vi "init.vi"(8 "error in (no error)":errorcluster, 11 "Counter in":refnum<class "Counter.lvclass">) -> (0 "error out":errorcluster, 3 "Counter out":refnum<class "Counter.lvclass">)   [LabVIEW 2014, in "Counter.lvclass"]
uses:
  Counter.lvclass
  Counter.lvclass/Counter.ctl
  Globals.vi
  <vilib>/DAQmx/create/channels.llb/DAQmx Create Channel (CI-Count Edges).vi
  <vilib>/DAQmx/configure/timing.llb/DAQmx Timing (Sample Clock).vi
  <resource>/objmgr/daqmx.rc
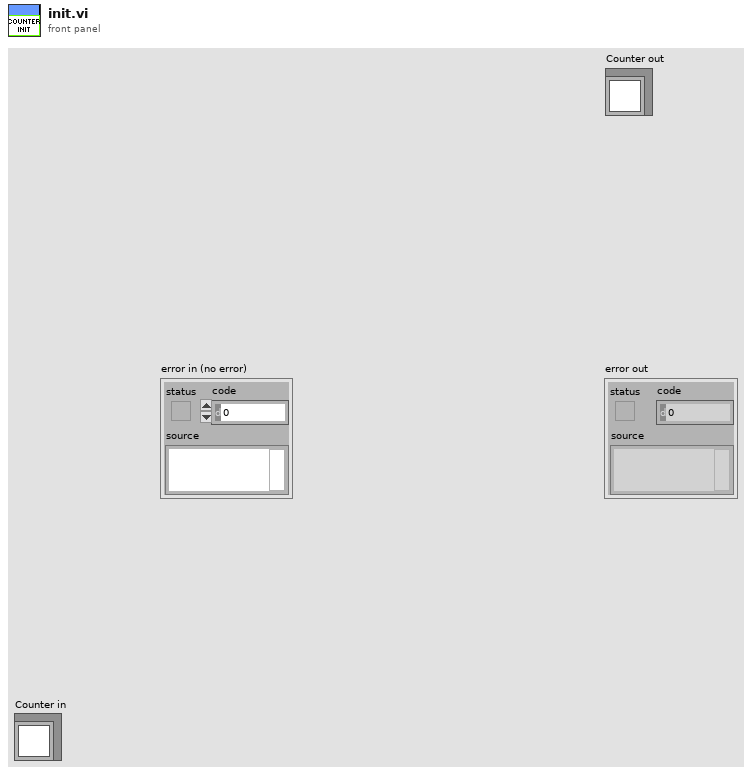
[diagram p1: front panel]
types:
  T1 = cluster{"counter source":tag, "clock source":tag, "clock rate (Hz)":dbl}[]
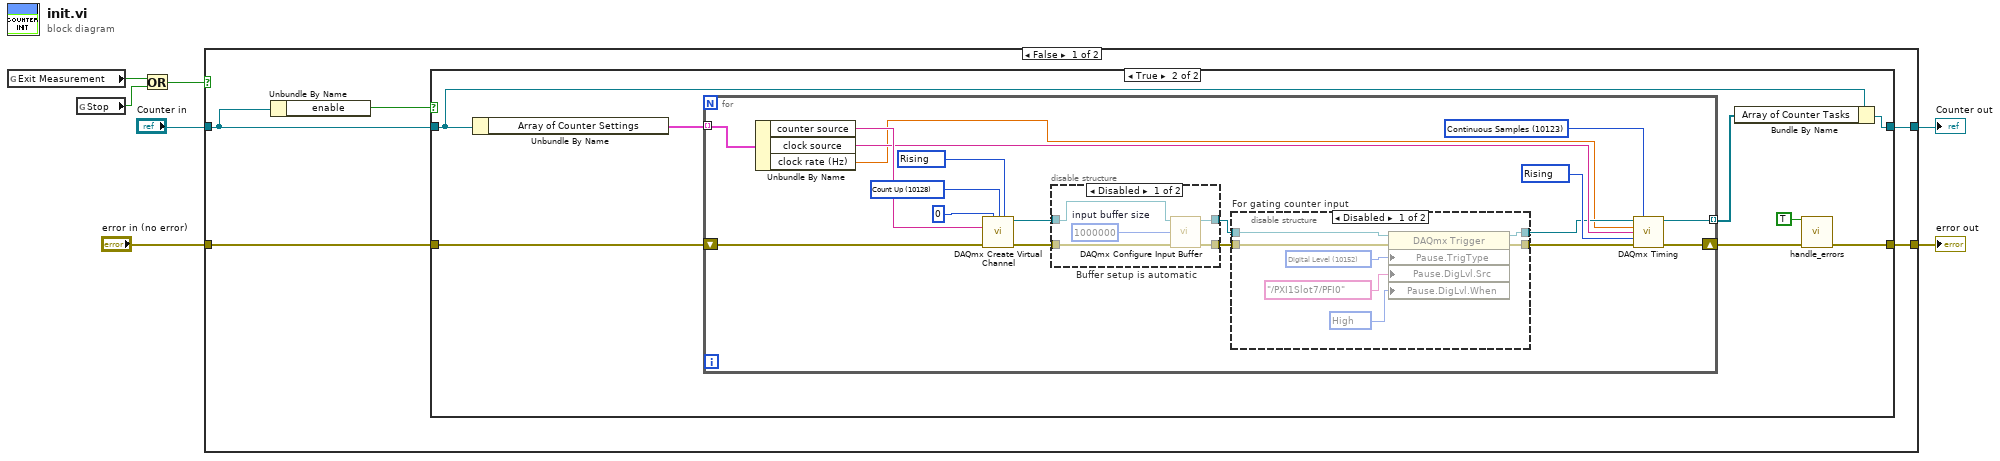
[diagram p0: block diagram]
diagram:
  n1 = global read "Globals.vi" "Exit Measurement"() -> (w4:bool)
  n2 = global read "Globals.vi" "Stop"() -> (w3:bool)
  n3 = Or(x=w4, y=w3) -> (x .or. y?=w2:bool)
  n4 = case shown="False" w2 {
    tunnel: [w11 w57] -> w7
    tunnel: [w10 w58] -> w5
    tunnel: "Counter in" -> [w8 w58]
    tunnel: "error in (no error)" -> [w9 w57]
    frame False {
      n5 = Unbundle By Name(w8) -> ("enable"=w12:bool)
      n6 = case shown="True" w12 {
        tunnel: w9 -> [w14 w22]
        tunnel: [w14 w15] -> w11
        tunnel: [w13 w20] -> w10
        tunnel: w8 -> [w13 w18]
        frame False {
        }
        frame True {
          n7 = Unbundle By Name(w18) -> ("Array of Counter Settings"=w19:T1)
          n8 = for {
            tunnel: w19 -> [w40] mode=indexing
            shift-right: [w36] -> w16
            shift-left: w22 -> [w39]
            tunnel: [w35] -> w21 mode=indexing
            w30 = 10280 items=["Rising"=10280, "Falling"=10171] ("active edge")
            w31 = 10123 items=["Finite Samples"=10178, "Continuous Samples"=10123, "Hardware Timed Single Point"=12522] ("sample mode")
            w32 = 10280 items=["Rising"=10280, "Falling"=10171] ("edge")
            w33 = 10128 items=["Count Up"=10128, "Count Down"=10124, "Externally Controlled"=10326] ("count direction")
            n9 = Unbundle By Name(w40) -> ("counter source"=w38:tag, "clock source"=w37:tag, "clock rate (Hz)"=w23:dbl)
            n10 = call-poly <vilib>:"DAQmx Create Virtual Channel.vi"("initial count"=u32 0, "count direction"=w33, "edge"=w32, "counter"=w38, "error in"=w39) -> ("task out"=w29:refnum<k21>, "error out"=w28:errorcluster)  [unwired: 5 in, 4 out]
            n11 = disable-structure "Buffer setup is automatic" shown="Disabled" {
              disable-tunnel: w29 -> [w54 w55]
              disable-tunnel: w28 -> [w53 w56]
              disable-tunnel: [w52 w56] -> w26
              disable-tunnel: [w51 w55] -> w27
              frame Disabled {
                w50 = u32 1000000  # input buffer size
                n12 = call <vilib>:"DAQmx Configure Input Buffer.vi"("task/channels in"=w54, "buffer size (in samples per channel)"=w50, "error in"=w53) -> ("task out"=w51:refnum<k21>, "error out"=w52:errorcluster)  [unwired: 11 out]
              }
              frame Enabled {
              }
            }
            n13 = disable-structure "For gating counter input" shown="Disabled" {
              disable-tunnel: w27 -> [w47 w48]
              disable-tunnel: w26 -> [w46 w49]
              disable-tunnel: [w42 w48] -> w25
              disable-tunnel: [w41 w49] -> w24
              frame Disabled {
                w43 = 10152 items=["Analog Level"=10101, "Analog Window"=10103, "Digital Level"=10152, "Digital Pattern"=10398, "None"=10230] ("Pause.TrigType")
                w45 = 10192 items=["High"=10192, "Low"=10214] ("Pause.DigLvl.When")
                n14 = property class="DAQmx Trigger"(reference=w47, error in=w46, "Pause.TrigType"=w43, "Pause.DigLvl.Src"=tag "/PXI1Slot7/PFI0", "Pause.DigLvl.When"=w45) -> (reference out=w42:refnum<k21>, error out=w41:errorcluster)
              }
              frame Enabled {
              }
            }
            n15 = call-poly <vilib>:"DAQmx Timing.vi"("task/channels in"=w25, "sample mode"=w31, "rate"=w23, "source"=w37, "active edge"=w30, "error in"=w24) -> ("task out"=w35:refnum<k21>, "error out"=w36:errorcluster)  [unwired: 1 in, 7 out]
          }
          n16 = Bundle By Name(cluster=w18, "Array of Counter Tasks"=w21) -> (w20:refnum<class "Counter.lvclass">)
          n17 = call "handle_errors.vi"("Exit Operation"=TRUE, "error in (no error)"=w16) -> ("error out"=w15:errorcluster)  [unwired: 13 in]
        }
      }
    }
    frame True {
    }
  }
  "error out" <- w7
  "Counter out" <- w5
